vi "CheckTreeTest.vi"() -> ()   [LabVIEW 2020]
uses:
  controls/DecisionTreeRecord.ctl
  controls/Player.ctl
  controls/Gameboard Data.ctl
  GetEquivalentKeysNumeric.vi
  MakeSquare.vi
  Flatten2DArray.vi
  <vilib>/Utility/error.llb/Error Cluster From Error Code.vi
  GetAllIsometriesOf2DArray.vi
panel:
  out "Passed?":bool[](array[boolean])
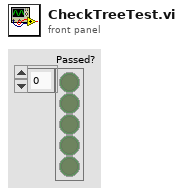
[diagram p1: front panel]
types:
  T1 = typedef "Gameboard Data.ctl" = enum16{"None", "Player 1", "Player 2"}[]
  T2 = typedef "DecisionTreeRecord.ctl" = cluster{"Status":T3, "GoodMoves":i8[], "MehMoves":i8[], "BadMoves":i8[]}
  T3 = typedef "Player.ctl" = enum16{"None", "Player 1", "Player 2"}
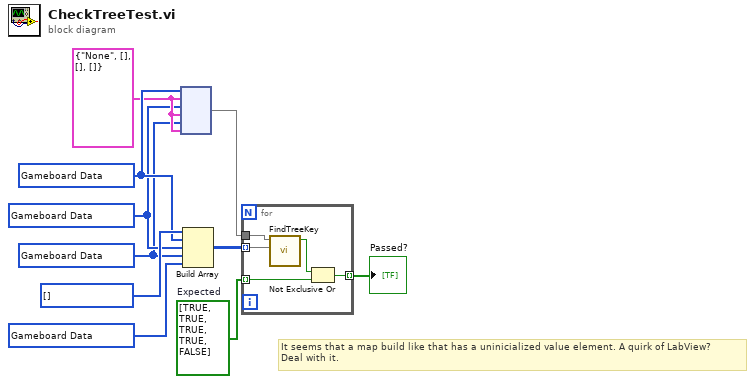
[diagram p0: block diagram]
diagram:
  w2 = bool[] [TRUE, TRUE, TRUE, TRUE, FALSE]  # Expected
  w3 = T1 [enum."Player 2", enum."None", enum."None", enum."None", enum."None", enum."None", enum."None", enum."None", enum."None"] items=["None", "Player 1", "Player 2"] ("Gameboard")
  w4 = T1 [enum."None", enum."None", enum."None", enum."Player 1", enum."None", enum."None", enum."None", enum."None", enum."None"] items=["None", "Player 1", "Player 2"] ("Gameboard")
  w5 = T1 [enum."Player 1", enum."None", enum."None", enum."None", enum."None", enum."None", enum."None", enum."None", enum."None"] items=["None", "Player 1", "Player 2"] ("Gameboard")
  w7 = T1 [enum."None", enum."None", enum."None", enum."None", enum."None", enum."None", enum."None", enum."None", enum."None"] items=["None", "Player 1", "Player 2"] ("Gameboard")
  w10 = T1 [] items=["None", "Player 1", "Player 2"] ("Gameboard")
  w6 = T2 {"Status"=enum."None", "GoodMoves"=[], "MehMoves"=[], "BadMoves"=[]} ("DecisionRecord")
  # "It seems that a map build like that has a uninicialized value element. A quirk of LabView?\nDeal with it."
  n1 = node(w7, w6, w5, w6, w4, w6) -> (w8:map{T1, T2})
  n2 = Build Array(w10, w7, w5, w4, w3) -> (w9:enum16{"None", "Player 1", "Player 2"}[][])
  n3 = for {
    tunnel: w8 -> [w15]
    tunnel: w9 -> [w14] mode=indexing
    tunnel: w2 -> [w12] mode=indexing
    tunnel: [w11] -> w1 mode=indexing
    n4 = call "FindTreeKey.vi"("Key"=w14, "Map"=w15) -> ("IsFound?"=w13:bool)  [unwired: 6 in, 3 out]
    n5 = Not Exclusive Or(1:w12, 2:w13) -> (0:w11:bool)
  }
  "Passed?" <- w1
